vi "test8.vi"() -> ()   [LabVIEW 2020]
uses:
  <vilib>/Platform/TimedLoop/XDataNode/timing_clust.ctl
  <vilib>/Platform/TimedLoop/XDataNode/nitl_modes.ctl
  <vilib>/Platform/TimedLoop/XDataNode/wakeup.ctl
  37583fcc-cec8-480d-a6d0-1da09da3d0dd.vi
  <vilib>/platform/TimedLoop/XDataNode/XDataNode.xnode
  <vilib>/Instr/_visa.llb/VISA Configure Serial Port (Instr).vi
  <vilib>/Platform/TimedLoop/XDataNode/XDNodeRunTimeDep.lvlib
panel:
  out "resulting string":string
  out "error out":errorcluster
  in  "VISA resource name":refnum<visa-resource-name>
  out "Distance 2":dbl
  out "Move Time 2":u32
  in  "Array":cluster{"x":dbl, "y":dbl}[](array[cluster])
  out "Tank":dbl(slide) scale=0.0..1.0
  out "Current XY":cluster{"X":dbl, "Y":dbl}
  out "XY Graph":cluster{dbl[], dbl[]}[](graph)
  in  "Stop":bool
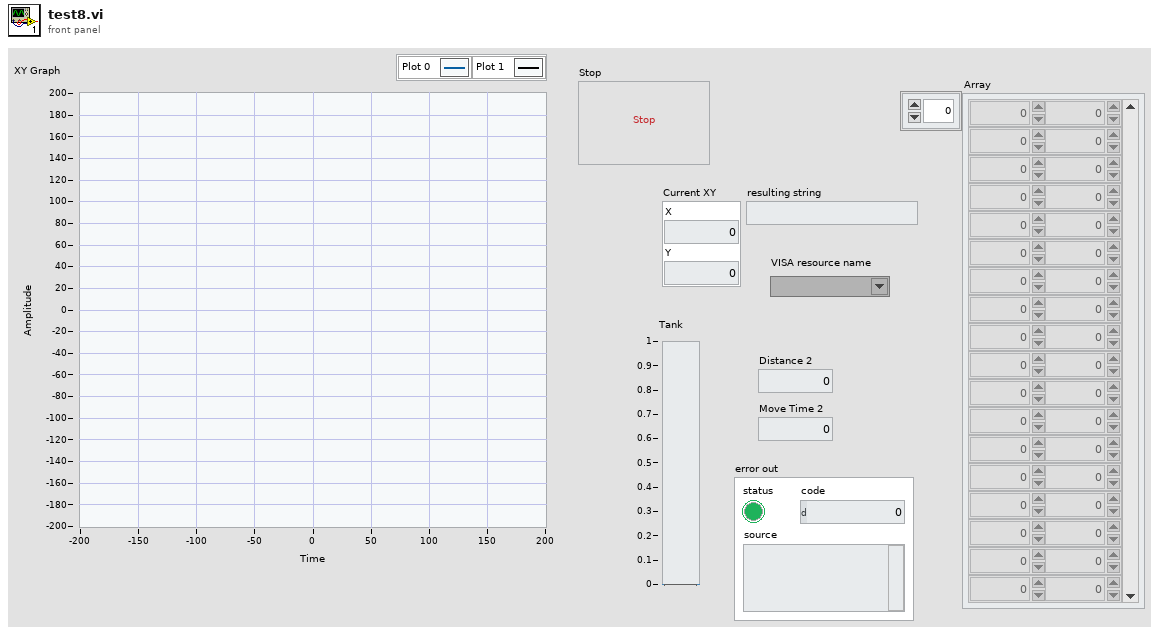
[diagram p1: front panel]
types:
  T1 = typedef "XDNodeRunTimeDep.lvlib/timing_clust.ctl" = cluster{"Expected End [f-1]":u64, "Actual End [f-1]":u64, "Finished Late? [f-1]":bool, "Expected End [i-1]":u64, "Actual End [i-1]":u64, "Finished Late? [i-1]":bool, "Expected Start [i]":u64, "Actual Start [i]":u64, "Expected Start [f]":u64, "Actual Start [f]":u64, "Source Name":string, "Structure Name":string, "Period":i64, "Deadline":i64, "Offset":i64, "Start":i64, "Priority":i32, "Timeout":i32, "Mode":T2, "Wakeup Reason":T3, "Error":errorcluster, "Source Type":string, "Secondary Source Type":string, "Global End Time":u64, "Global Start Time":u64, "Frame Duration":u64, "Iteration Duration":u64, "Assigned CPU":i32, "I/O Scan Engine Mode":u32}
  T2 = typedef "XDNodeRunTimeDep.lvlib/nitl_modes.ctl" = enum32{"No Change", "Process missed periods, maintain original phase", "Discard missed periods, maintain original phase", "Process missed periods, ignore original phase", "Discard missed periods, ignore original phase"}
  T3 = typedef "XDNodeRunTimeDep.lvlib/wakeup.ctl" = enum32{"Normal", "Aborted", "Asynchronous wakeup", "Timing source error", "Timed loop error", "Timeout"}
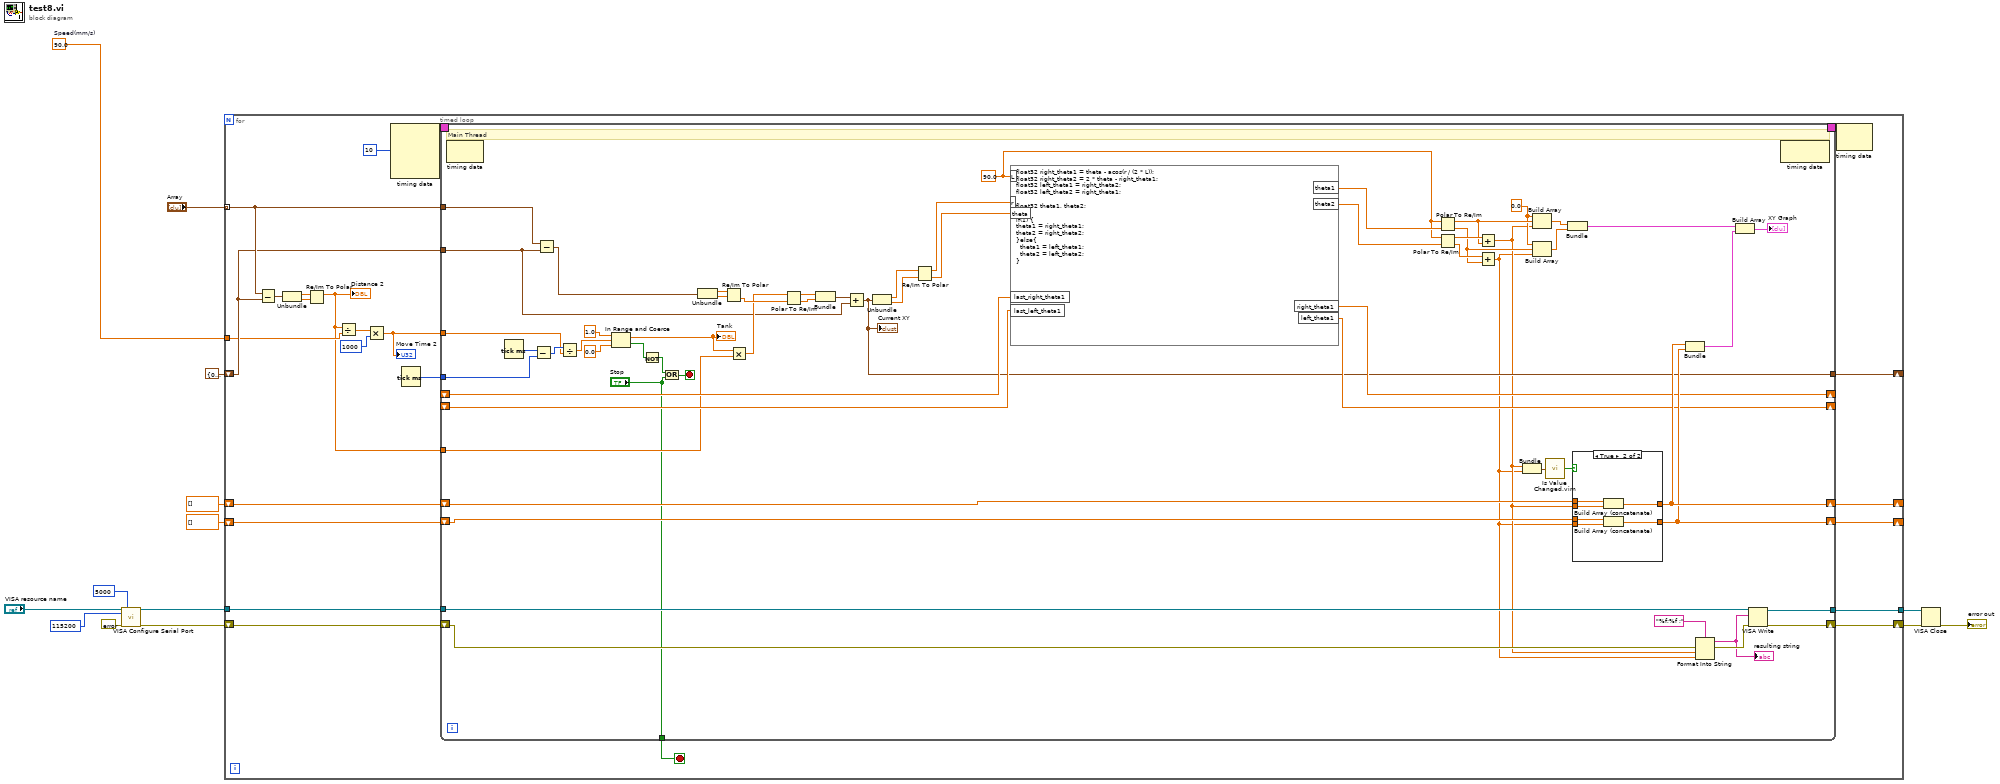
[diagram p0: block diagram]
diagram:
  w12 = 90.0  # Speed(mm/s)
  n1 = call-poly "VISA Configure Serial Port"("VISA resource name"="VISA resource name", "timeout (10sec)"=u32 5000, "baud rate (9600)"=u32 115200, "error in (no error)"=errorcluster {"status"=FALSE, "code"=0, "source"=""}) -> ("VISA resource name out"=w4:refnum<visa-resource-name>, "error out"=w5:errorcluster)  [unwired: 10 in]
  n2 = for {
    tunnel: "Array" -> [w29] mode=indexing
    shift-right: [w35] -> _
    shift-left: cluster{dbl, dbl} {0.0, 0.0} -> [w28]
    tunnel: w12 -> [w27]
    shift-right: [w22] -> _
    shift-left: dbl[] [] -> [w23]
    shift-right: [w21] -> _
    shift-left: dbl[] [] -> [w20]
    shift-right: [w17] -> w3
    shift-left: w5 -> [w19]
    tunnel: w4 -> [w18]
    tunnel: [w16] -> w2
    stop <- w15 stop-if-true
    n3 = Subtract(x=w29, y=w28) -> (x-y=w32:cluster{dbl, dbl})
    n4 = Unbundle(w32) -> (w31:dbl, w30:dbl)
    n5 = Re/Im To Polar(2:w30, 3:w31) -> (1:w25:dbl)  [unwired: 1 out]
    "Distance 2" <- w25
    n6 = Divide(x=w25, y=w27) -> (x/y=w33:dbl)
    n7 = Multiply(x=w33, y=u32 1000 ("millisecond timer value")) -> (x*y=w26:dbl)
    "Move Time 2" <- w26
    n8 = node-c288(i64 10 ("Period")) -> (w38:T1)  [unwired: 3 in]
    n9 = Tick Count (ms)() -> (millisecond timer value=w24:u32)
    n10 = timed-loop {
      timing: w38 -> [_]
      timing-out: [_] -> w37
      shift-right: [w70] -> w22
      shift-left: w23 -> [w75]
      shift-right: [w69] -> w21
      shift-left: w20 -> [w74]
      shift-right: [w60] -> _
      shift-left: _ -> [w59]
      shift-right: [w61] -> _
      shift-left: _ -> [w58]
      tunnel: w29 -> [w56]
      tunnel: [w55] -> w35
      tunnel: w28 -> [w54]
      tunnel: w26 -> [w53]
      tunnel: w25 -> [w52]
      tunnel: w24 -> [w51]
      shift-right: [w45] -> w17
      shift-left: w19 -> [w47]
      tunnel: w18 -> [w46]
      tunnel: [w44] -> w16
      tunnel: ["Stop"] -> w15
      stop <- w40 stop-if-true
      w79 = 0.0 ("element")
      w76 = 90.0 ("input variable")
      # "Main Thread"
      n11 = node-c288() -> ()  [unwired: 1 in, 1 out]
      n12 = Tick Count (ms)() -> (millisecond timer value=w98:u32)
      n13 = Subtract(x=w98, y=w51) -> (x-y=w66:u32)
      n14 = Subtract(x=w56, y=w54) -> (x-y=w97:cluster{dbl, dbl})
      n15 = Divide(x=w66, y=w53) -> (x/y=w65:dbl)
      n16 = In Range and Coerce(upper limit=1.0 ("lower limit"), x=w65, lower limit=0.0) -> (coerced(x)=w62:dbl, In Range?=w57:bool)
      "Tank" <- w62
      n17 = Not(x=w57) -> (.not. x?=w41:bool)
      n18 = Or(x=w41, y="Stop") -> (x .or. y?=w40:bool)
      n19 = Unbundle(w97) -> (w96:dbl, w95:dbl)
      n20 = Re/Im To Polar(2:w95, 3:w96) -> (0:w94:dbl)  [unwired: 1 out]
      n21 = Multiply(x=w62, y=w52) -> (x*y=w87:dbl)
      n22 = Polar To Re/Im(2:w94, 3:w87) -> (0:w92:dbl, 1:w93:dbl)
      n23 = Bundle(w93, w92) -> (w91:cluster{dbl, dbl})  [unwired: 1 in]
      n24 = Add(x=w91, y=w54) -> (x+y=w55:cluster{dbl, dbl})
      "Current XY" <- w55
      n25 = Unbundle(w55) -> (w90:dbl, w89:dbl)
      n26 = Re/Im To Polar(2:w89, 3:w90) -> (0:w88:dbl, 1:w86:dbl)
      n27 = formula code="float32 right_theta1 = theta - acos(r / (2 * L));\nfloat32 right_theta2 = 2 * theta - right_theta1;\nfloat32 left_theta1 = right_theta2;\nfloat32 left_theta2 = right_theta1;\n\nfloat32 theta1, theta2;\n\nif(1) {\ntheta1 = right_theta1;\ntheta2 = right_theta2;\n}else{\n  theta1 = left_theta1;\n  theta2 = left_theta2;\n}"("r"=w86, "theta"=w88, "L"=w76, "last_right_theta1"=w59, "last_left_theta1"=w58) -> ("theta1"=w78:sgl, "theta2"=w77:sgl, "right_theta1"=w60:sgl, "left_theta1"=w61:sgl)
      n28 = Polar To Re/Im(2:w78, 3:w76) -> (0:w82:dbl, 1:w83:dbl)
      n29 = Polar To Re/Im(2:w77, 3:w76) -> (0:w84:dbl, 1:w85:dbl)
      n30 = Add(x=w85, y=w83) -> (x+y=w43:dbl)
      n31 = Add(x=w84, y=w82) -> (x+y=w42:dbl)
      n32 = Bundle(w43, w42) -> (w73:cluster{dbl, dbl})  [unwired: 1 in]
      n33 = Build Array(w79, w83, w43) -> (w81:dbl[])
      n34 = Build Array(w79, w82, w42) -> (w80:dbl[])
      n35 = call "Is Value Changed.vim"("value"=w73) -> ("changed or first call?"=w72:bool)
      n36 = Bundle(w81, w80) -> (w71:cluster{dbl[], dbl[]})  [unwired: 1 in]
      n37 = case shown="True" w72 {
        tunnel: w43 -> [_ w106]
        tunnel: w42 -> [_ w105]
        tunnel: [w100 w104] -> w70
        tunnel: [w99 w103] -> w69
        tunnel: w75 -> [w100 w102]
        tunnel: w74 -> [w99 w101]
        frame False {
        }
        frame True {
          n38 = Build Array (concatenate)(w102, w106) -> (w104:dbl[])
          n39 = Build Array (concatenate)(w101, w105) -> (w103:dbl[])
        }
      }
      n40 = Bundle(w70, w69) -> (w68:cluster{dbl[], dbl[]})  [unwired: 1 in]
      n41 = Format Into String(format string="%f;%f ;", error in=w47, w43, w42) -> (resulting string=w48:string, error out=w49:errorcluster)  [unwired: 1 in]
      "resulting string" <- w48
      n42 = Build Array(w71, w68) -> (→"XY Graph":cluster{dbl[], dbl[]}[])
      n43 = VISA Write(VISA resource name=w46, write buffer=w48, error in (no error)=w49) -> (VISA resource name out=w44:refnum<visa-resource-name>, error out=w45:errorcluster)  [unwired: 1 out]
      n44 = node-c288() -> ()  [unwired: 1 in, 1 out]
    }
    n45 = node-c288(w37) -> ()  [unwired: 1 out]
  }
  n46 = VISA Close(VISA resource name=w2, error in (no error)=w3) -> (error out=→"error out":errorcluster)
